vi "MODE_SETS.vi"(9 "Mode":u8=35 format="%.0b", 11 "Python in":string) -> (3 "Python out":string)   [LabVIEW 2016]
panel:
  out "bytes added":u8[](array[numeric])=[64, 35, 0] format="%.0b"
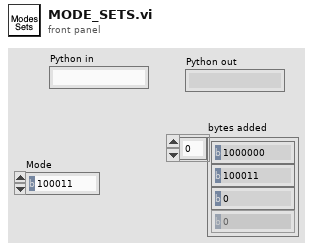
[diagram p1: front panel]
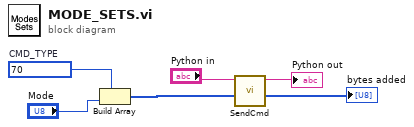
[diagram p0: block diagram]
diagram:
  w3 = u8 70  # CMD_TYPE
  n1 = Build Array(w3, "Mode") -> (w1:u8[])
  n2 = call "SendCmd.vi"("Array In"=w1, "Python in"="Python in") -> ("Array Sent"=→"bytes added":u8[], "Python out"=→"Python out":string)  [unwired: 8 in]
